vi "VIE.Module.Queued Message Handler.dequeue.State.QueuedMessageHandler.vi"(8 "error in (no error)":errorcluster, 9 "Timeout (0ms)":i32, 10 "QueuedMessageHandler.dqGOOPClass (in)":T1) -> (0 "error out":errorcluster, 1 "State Dequeued":string, 2 "QueuedMessageHandler.dqGOOPClass (out)":T1)   [LabVIEW 2010, in "VIE.Module.Queued Message Handler.QueuedMessageHandler.dqGOOPClass.lvlib"]
uses:
  VIE.Module.Queued Message Handler.QueuedMessageHandler.dqGOOPClass.lvlib
  VIE.Module.Queued Message Handler.dqClass_ObjectReference.ctl
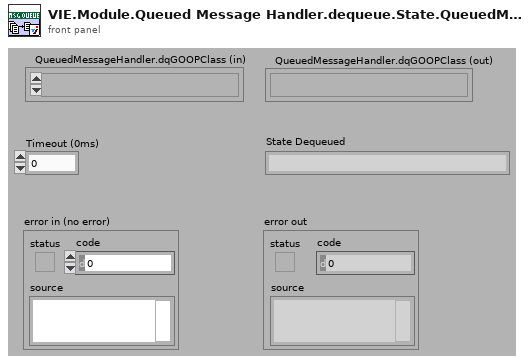
[diagram p1: front panel]
types:
  T1 = typedef "VIE.Module.Queued Message Handler.QueuedMessageHandler.dqGOOPClass.lvlib/VIE.Module.Queued Message Handler.dqClass_ObjectReference.ctl" = refnum<k1>
  T2 = typedef "VIE.Module.Queued Message Handler.QueuedMessageHandler.dqGOOPClass.lvlib/VIE.Module.Queued Message Handler.dqClass_ObjectData.ctl" = cluster{"Message Queue":refnum<queue>, "Log File Refnum":refnum<file>}
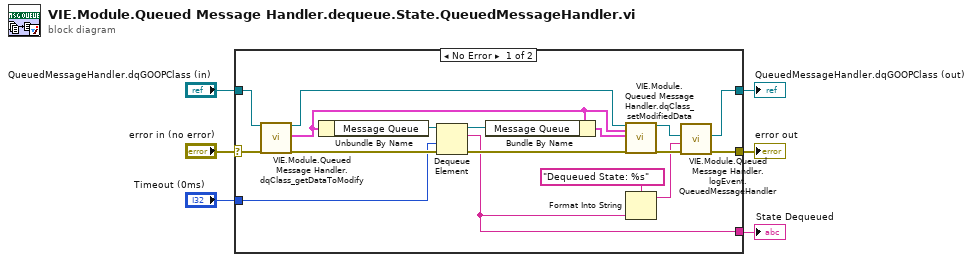
[diagram p0: block diagram]
diagram:
  n1 = case shown="No Error" "error in (no error)" {
    selector: "error in (no error)" -> [w18 w25]
    tunnel: [w21 w25] -> w5
    tunnel: [w20 w24] -> w4
    tunnel: "QueuedMessageHandler.dqGOOPClass (in)" -> [w16 w24]
    tunnel: [w10 _] -> w2
    tunnel: "Timeout (0ms)" -> [w7 _]
    frame No Error {
      n2 = call "VIE.Module.Queued Message Handler.dqClass_getDataToModify.vi"("reference"=w16, "error in (no error)"=w18) -> ("duplicate reference"=w13:T1, "data"=w11:T2, "error out"=w17:errorcluster)  [unwired: 14 in, 1 out]
      n3 = Unbundle By Name(w11) -> ("Message Queue"=w23:refnum<queue>)
      n4 = Dequeue Element(queue=w23, timeout in ms (-1)=w7, error in (no error)=w17) -> (queue out=w22:refnum<queue>, element=w10:string, error out=w15:errorcluster)  [unwired: 1 out]
      n5 = Bundle By Name(cluster=w11, "Message Queue"=w22) -> (w12:T2)
      n6 = call "VIE.Module.Queued Message Handler.dqClass_setModifiedData.vi"("reference"=w13, "data (unmodified)"=w11, "data"=w12, "error in (no error)"=w15) -> ("duplicate reference"=w8:T1, "error out"=w14:errorcluster)  [unwired: 14 in]
      n7 = Format Into String(format string="Dequeued State: %s", w10) -> (resulting string=w9:string)  [unwired: 2 in, 1 out]
      n8 = call "VIE.Module.Queued Message Handler.logEvent.QueuedMessageHandler.vi"("error in (no error)"=w14, "Event to Log"=w9, "QueuedMessageHandler.dqGOOPClass (in)"=w8) -> ("error out"=w21:errorcluster, "QueuedMessageHandler.dqGOOPClass (out)"=w20:T1)  [unwired: 7 in]
    }
    frame Error {
    }
  }
  "error out" <- w5
  "QueuedMessageHandler.dqGOOPClass (out)" <- w4
  "State Dequeued" <- w2
